vi "WriteLine to File.vi"(8 "error in":errorcluster, 10 "Line To Write":string, 11 "path in":path) -> (0 "error out":errorcluster, 3 "path out":path)   [LabVIEW 2016]
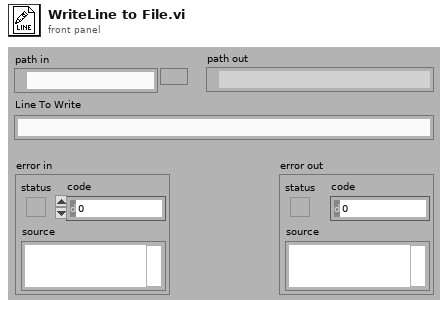
[diagram p1: front panel]
types:
  T1 = enum16{"open", "replace", "create", "open or create", "replace or create", "replace or create with confirmation"}
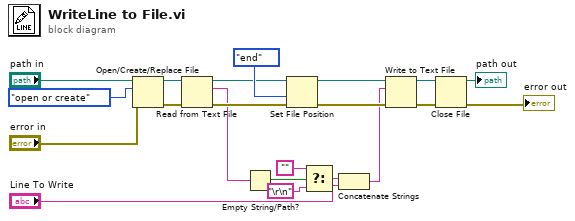
[diagram p0: block diagram]
diagram:
  n1 = Open/Create/Replace File(file path (use dialog)="path in", error in="error in", operation (0:open)=T1."open or create") -> (refnum out=w18:refnum<file>, error out=w17:errorcluster)  [unwired: 3 in, 1 out]
  n2 = Read from Text File(file (use dialog)=w18, error in=w17) -> (refnum out=w12:refnum<file>, text=w5:string, error out=w14:errorcluster)  [unwired: 2 in, 1 out]
  n3 = Empty String/Path?(string/path=w5) -> (empty?=w13:bool)
  n4 = Set File Position(refnum=w12, from (0:start)=enum16{"start", "end", "current"}."end", error in=w14) -> (refnum out=w11:refnum<file>, error out=w10:errorcluster)  [unwired: 1 in]
  n5 = Select(t="", s=w13, f="\r\n") -> (s? t:f=w9:string)
  n6 = Concatenate Strings(w9, "Line To Write") -> (w7:string)
  n7 = Write to Text File(file (use dialog)=w11, text=w7, error in=w10) -> (refnum out=w20:refnum<file>, error out=w19:errorcluster)  [unwired: 1 in, 1 out]
  n8 = Close File(refnum=w20, error in=w19) -> (path=→"path out":path, error out=→"error out":errorcluster)
